vi "ServerNetworkInterface.vi"() -> ()   [LabVIEW 2025]
uses:
  ServerNetworkInterfaceGlobalVariables.vi
panel:
  out "recv error":errorcluster
  out "send error":errorcluster
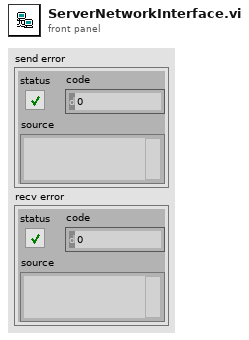
[diagram p1: front panel]
types:
  T1 = cluster{"Data":string, "Address":u32, "Port":u16}
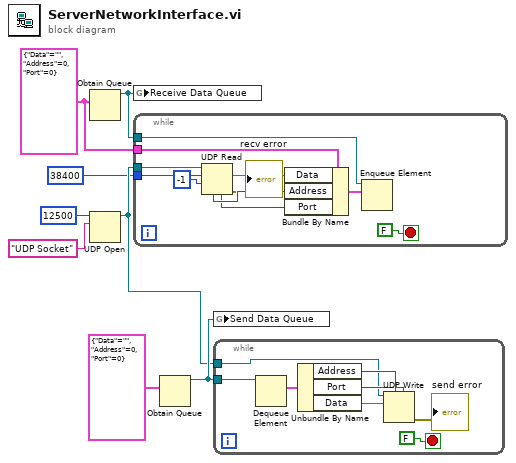
[diagram p0: block diagram]
diagram:
  w6 = T1 {"Data"="", "Address"=0, "Port"=0}
  n1 = Obtain Queue(element data type=w6) -> (queue out=w5:refnum<queue>)  [unwired: 4 in, 2 out]
  n2 = UDP Open(10:"UDP Socket" ("service name"), 11:u16 12500 ("port")) -> (port=w2:refnum<k16>)  [unwired: 3 in, 2 out]
  n3 = global write "ServerNetworkInterfaceGlobalVariables.vi" "Receive Data Queue"(w5) -> ()
  n4 = while {
    tunnel: w2 -> [w19]
    tunnel: w5 -> [w18]
    tunnel: w6 -> [w16]
    tunnel: 38400 ("max size (548)") -> [w10]
    stop <- FALSE stop-if-true
    n5 = UDP Read(connection ID=w19, max size (548)=w10, timeout ms (25000)=-1) -> (data out=w17:string, error out=→"recv error":errorcluster, 4:w14:u16, 6:w15:u32)  [unwired: 1 in, 1 out]
    n6 = Bundle By Name(cluster=w16, "Data"=w17, "Address"=w15, "Port"=w14) -> (w13:T1)
    n7 = Enqueue Element(queue=w18, element=w13) -> ()  [unwired: 2 in, 3 out]
  }
  n8 = Obtain Queue(element data type=T1 {"Data"="", "Address"=0, "Port"=0}) -> (queue out=w3:refnum<queue>)  [unwired: 4 in, 2 out]
  n9 = global write "ServerNetworkInterfaceGlobalVariables.vi" "Send Data Queue"(w3) -> ()
  n10 = while {
    tunnel: w3 -> [w25]
    tunnel: w2 -> [w21]
    stop <- FALSE stop-if-true
    n11 = Dequeue Element(queue=w25) -> (element=w27:T1)  [unwired: 2 in, 3 out]
    n12 = Unbundle By Name(w27) -> ("Address"=w24:u32, "Port"=w23:u16, "Data"=w22:string)
    n13 = UDP Write(address=w24, port or service name=w23, connection ID=w21, data in=w22) -> (error out=→"send error":errorcluster)  [unwired: 2 in, 1 out]
  }
